vi "Read Swich Rule and Polarity.vi"(0 "class data in":refnum<class "MB_ENGINE.lvclass">, 5 "SW":u16, 11 "error in (no error)":errorcluster) -> (4 "class data out":refnum<class "MB_ENGINE.lvclass">, 6 "Switch Rule and Polarity":T1, 15 "error out":errorcluster)   [LabVIEW 2019, in "MB_ENGINE.lvclass"]
uses:
  MB_ENGINE.lvclass
  Switch Rule and Polarity.ctl
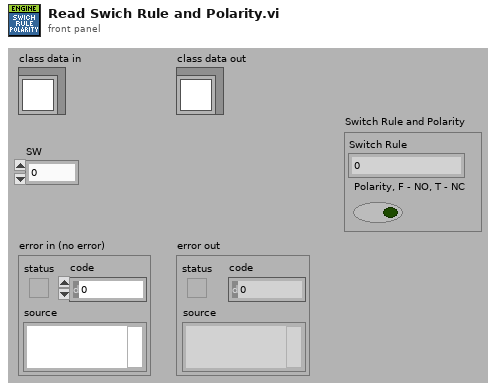
[diagram p1: front panel]
types:
  T1 = typedef "MB_ENGINE.lvclass/Switch Rule and Polarity.ctl" = cluster{"Switch Rule":u8, "Polarity, F - NO, T - NC":bool}
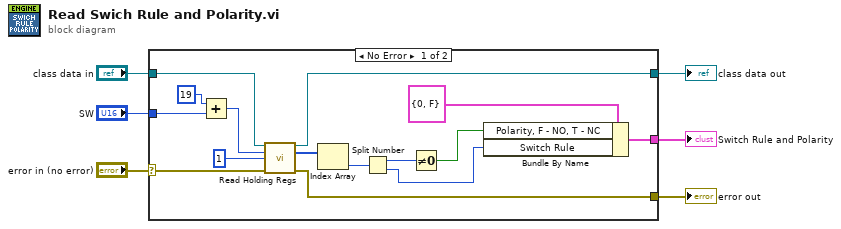
[diagram p0: block diagram]
diagram:
  n1 = case shown="No Error" "error in (no error)" {
    selector: "error in (no error)" -> [w20 w23]
    tunnel: [w17 w23] -> w5
    tunnel: "class data in" -> [w21 w22]
    tunnel: [w7 w22] -> w3
    tunnel: "SW" -> [w15 _]
    tunnel: [w9 _] -> w1
    frame No Error {
      n2 = Add(x=u16 19 ("starting address"), y=w15) -> (x+y=w16:u16)
      n3 = call-dynamic "Read Holding Regs.vi"("reference in"=w21, "starting address"=w16, "number of inputs"=u16 1, "error in (no error)"=w20) -> ("reference out"=w7:refnum<class "MB_ENGINE.lvclass">, "register values"=w8:u16[], "error out"=w17:errorcluster)  [unwired: 9 in]
      n4 = Index Array(array=w8) -> (element=w13:u16)  [unwired: 1 in]
      n5 = Split Number(x=w13) -> (hi(x)=w11:u8, lo(x)=w12:u8)
      n6 = Not Equal To 0?(x=w11) -> (x != 0?=w10:bool)
      n7 = Bundle By Name(cluster=T1 {"Switch Rule"=0, "Polarity, F - NO, T - NC"=FALSE} ("Cluster"), "Polarity, F - NO, T - NC"=w10, "Switch Rule"=w12) -> (w9:T1)
    }
    frame Error {
    }
  }
  "error out" <- w5
  "class data out" <- w3
  "Switch Rule and Polarity" <- w1
